vi "Actor Core.vi"(8 "error in":errorcluster, 11 "Guest Manager UI in":refnum<class "Guest Manager UI.lvclass">) -> (0 "error out":errorcluster, 3 "Actor out":refnum<class "Actor.lvclass">)   [LabVIEW 2023, in "Guest Manager UI.lvlib" / "Guest Manager UI.lvclass"]
doc: "(<B>Filename</B>: Actor Framework.lvlib:Actor.lvclass:Actor Core.vi)\n\nReceives messages to the actor, reacts to them, and initiates any error handling that may shut the actor down.\n\nDescendant classes may override this VI to append parallel tasks for the actor to complete while it handles messages. Overrides use the Call Parent Class Method node."
uses:
  Guest Manager UI.lvclass
  C:/Users/bhaghyaraj/Trainings/NI Actor Framework/SDLC/UI Base/UI Base/UI Base.lvclass
  C:/Program Files/National Instruments/LabVIEW 2023/vi.lib/ActorFramework/Actor/Actor.lvclass
  <vilib>/ActorFramework/Actor/Actor.lvclass
  Guest Manager UI.lvclass/Guest Manager UI.ctl
  <vilib>/ActorFramework/Actor/Actor.lvclass/Actor.ctl
  <vilib>/ActorFramework/Message Enqueuer/Message Enqueuer.lvclass/Message Enqueuer.ctl
  Guest Manager UI Messages/Check Guest History Msg/Check Guest History Msg.lvclass/Check Guest History Msg.ctl
  Guest Manager UI Messages/Fetch Rooms List and Size Limits Msg/Fetch Rooms List and Size Limits Msg.lvclass/Fetch Rooms List and Size Limits Msg.ctl
  Guest Manager UI Messages/Fetch Room Details Msg/Fetch Room Details Msg.lvclass/Fetch Room Details Msg.ctl
  <vilib>/ActorFramework/Message Enqueuer/Enqueue.vi
  <vilib>/ActorFramework/Message Enqueuer/Init from Existing Queue.vi
  <vilib>/ActorFramework/Stop Msg/Stop Msg.lvclass
  C:/Program Files/National Instruments/LabVIEW 2023/vi.lib/ActorFramework/Message/Message.lvclass
  Guest Manager UI Messages/Check Guest History Msg/Check Guest History Msg.lvclass
  Guest Manager UI Messages/Fetch Rooms List and Size Limits Msg/Fetch Rooms List and Size Limits Msg.lvclass
  Guest Manager UI Messages/Request Check-In Msg/Request Check-In Msg.lvclass
  Guest Manager UI Messages/Fetch Room Details Msg/Fetch Room Details Msg.lvclass
  Guest Manager UI Messages/Request Check-Out Msg/Request Check-Out Msg.lvclass
  Guest Manager UI Messages/Fetch Room Sizes Msg/Fetch Room Sizes Msg.lvclass
  <vilib>/ActorFramework/Message Priority Queue/Priority Enqueue.vi
  <vilib>/ActorFramework/Message Enqueuer/Message Enqueuer.lvclass
  UI Base/UI Base/UI Base.lvclass
  Utilities/Utilities.lvlib
panel:
  in  "Operation":enum32{"Check-In", "Check-Out"}(tab)
  in  "Children":u32=1 min=1
  in  "Primary Guest Name In":string caption="Primary Guest Name"
  in  "Guest Contact Number In":string caption="Guest Contact Number"
  in  "Room Size":u16(ring) items=["Suite (Non-AC)"]
  in  "Room Number In":u16(ring) caption="Room Number" items=["305"]
  in  "Adults":u32=1 min=1
  in  "Check-In":bool
  in  "Check-Out":bool
  out "Bill Summary":string
  out "Guest Contact Number Out":string caption="Guest Contact Number"
  out "Primary Guest Name Out":string caption="Primary Guest Name"
  out "Room Number Out":string caption="Room Number"
  # "Guest Check-In"
  # "Guest Check-Out"
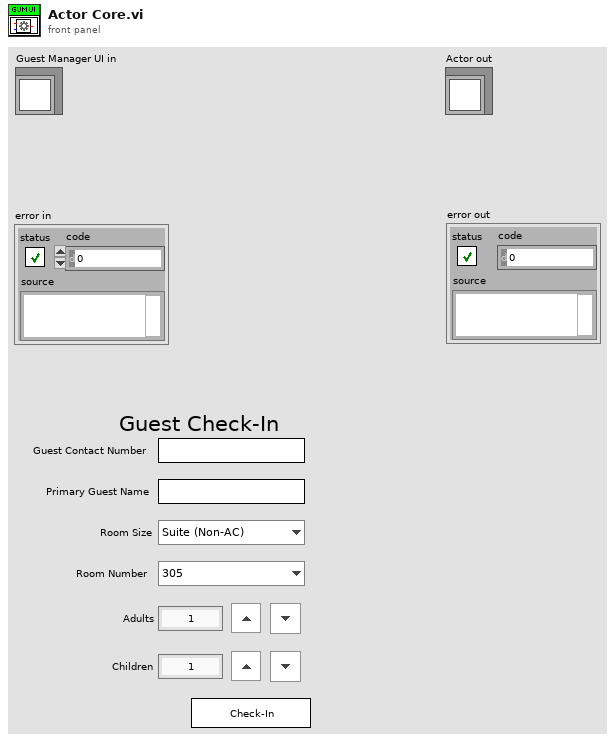
[diagram p1: front panel]
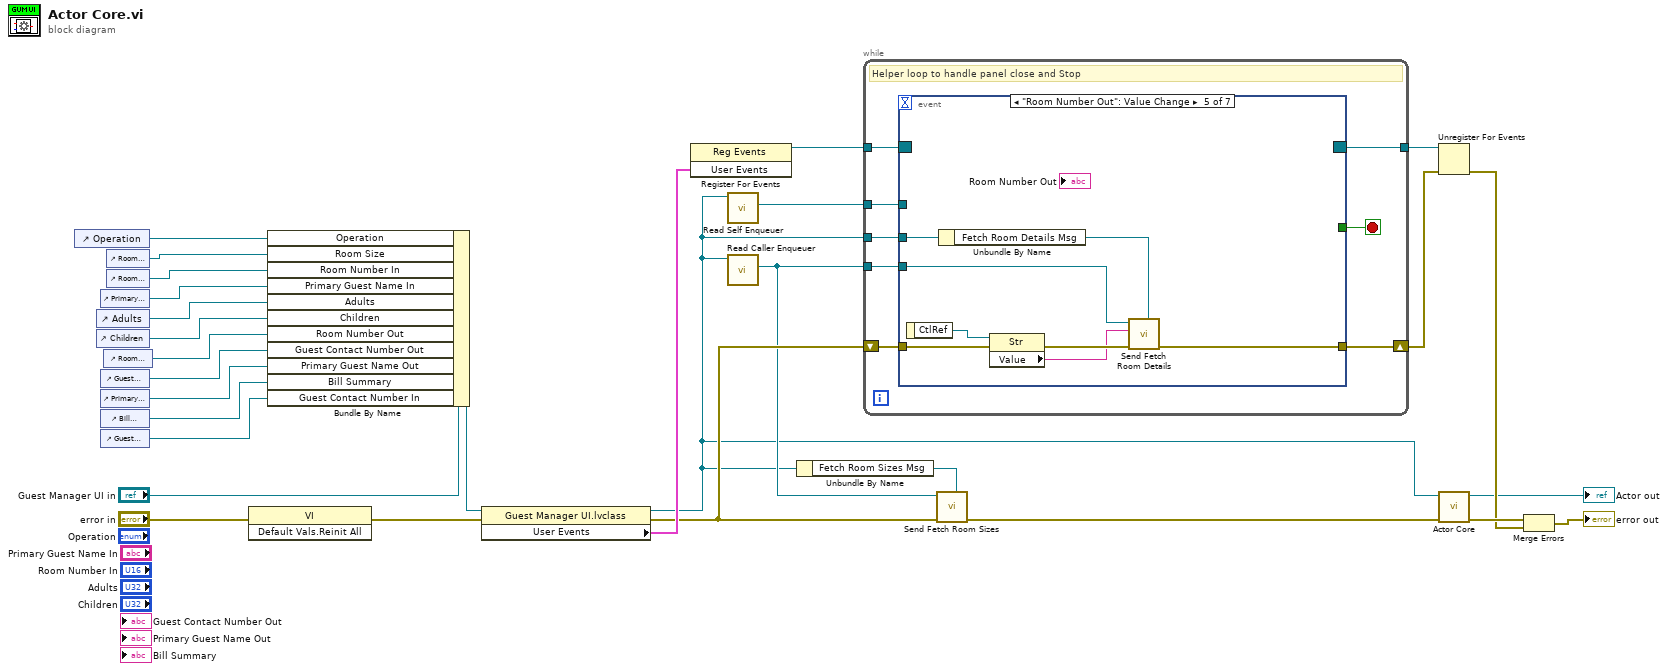
[diagram p0: block diagram]
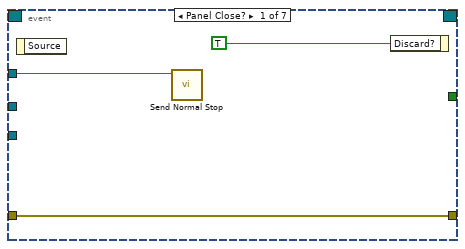
[diagram p2: hidden frame]
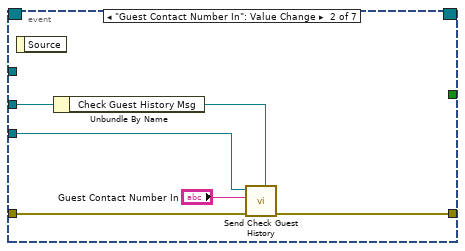
[diagram p3: hidden frame]
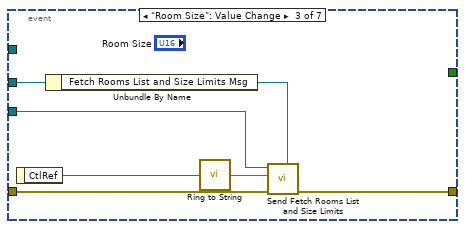
[diagram p4: hidden frame]
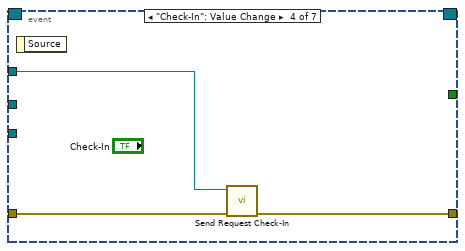
[diagram p5: hidden frame]
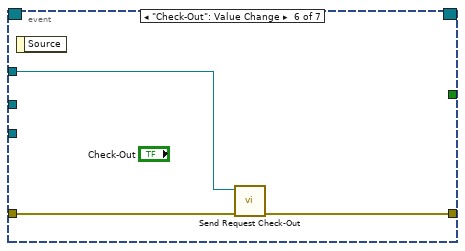
[diagram p6: hidden frame]
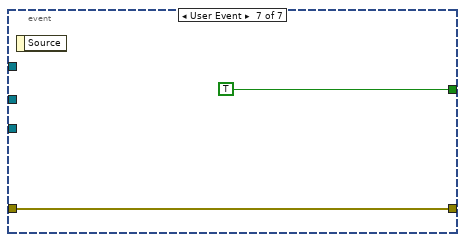
[diagram p7: hidden frame]
diagram:
  n1 = control-ref of="Operation"() -> (w17:refnum<vi>)
  n2 = control-ref of="Adults"() -> (w13:refnum<vi>)
  n3 = control-ref of="Children"() -> (w3:refnum<vi>)
  n4 = control-ref of="Primary Guest Name In"() -> (w14:refnum<vi>)
  n5 = control-ref of="Guest Contact Number Out"() -> (w11:refnum<vi>)
  n6 = control-ref of="Primary Guest Name Out"() -> (w10:refnum<vi>)
  n7 = control-ref of="Bill Summary"() -> (w9:refnum<vi>)
  n8 = control-ref of="Guest Contact Number In"() -> (w2:refnum<vi>)
  n9 = control-ref of="Room Number Out"() -> (w12:refnum<vi>)
  n10 = control-ref of="Room Size"() -> (w16:refnum<vi>)
  n11 = control-ref of="Room Number In"() -> (w15:refnum<vi>)
  n12 = invoke class="VI" method="Default Vals.Reinit All"(error in="error in") -> (error out=w1:errorcluster)  [unwired: 2 in, 2 out]
  n13 = Bundle By Name(cluster="Guest Manager UI in", "Operation"=w17, "Room Size"=w16, "Room Number In"=w15, "Primary Guest Name In"=w14, "Adults"=w13, "Children"=w3, "Room Number Out"=w12, "Guest Contact Number Out"=w11, "Primary Guest Name Out"=w10, "Bill Summary"=w9, "Guest Contact Number In"=w2) -> (w18:refnum<class "Guest Manager UI.lvclass">)
  n14 = property class="Guest Manager UI.lvclass"(reference=w18, error in=w1) -> (reference out=w5:refnum<class "Guest Manager UI.lvclass">, error out=w8:errorcluster, "User Events"=w25:cluster{"Stop":refnum<user-event>})
  n15 = register-events(w25) -> (reference out=w27:refnum<event-registration>)  [unwired: 2 in, 1 out]
  n16 = call <vilib>:"Read Self Enqueuer.vi"("Actor"=w5) -> ("Self Enqueuer"=w26:refnum<class "Message Enqueuer.lvclass">)  [unwired: 10 in]
  n17 = call <vilib>:"Read Caller Enqueuer.vi"("Actor"=w5) -> ("Caller Enqueuer"=w6:refnum<class "Message Enqueuer.lvclass">)  [unwired: 10 in]
  n18 = Unbundle By Name(w5) -> ("Fetch Room Sizes Msg"=w4:refnum<class "Fetch Room Sizes Msg.lvclass">)
  n19 = while {
    tunnel: w26 -> [w37]
    tunnel: w27 -> [w36]
    tunnel: [w34] -> w28
    tunnel: w6 -> [w33]
    tunnel: w5 -> [w32]
    shift-right: [w30] -> w23
    shift-left: w8 -> [w31]
    stop <- w35 stop-if-true
    # "Helper loop to handle panel close and Stop"
    n20 = event shown="[4] \"Room Number Out\": Value Change" {
      selector: w36 -> [_ _ _ _ _ _ _]
      dyn-events: [_ _ _ _ _ _ _] -> w34
      timeout: _ -> [_ _ _ _ _ _ _]
      tunnel: w37 -> [w39 _ _ w54 _ w65 _]
      tunnel: [_ _ _ _ _ _ TRUE] -> w35
      tunnel: w33 -> [_ w44 w51 _ w60 _ _]
      tunnel: w32 -> [_ w42 w50 _ w62 _ _]
      tunnel: w31 -> [w38 w46 w53 w56 w64 w67 w68]
      tunnel: [w38 w45 w52 w55 w63 w66 w68] -> w30
      event Panel Close? {
        n21 = event-data() -> ()  [unwired: 1 in, 1 out]
        n22 = call <vilib>:"Send Normal Stop.vi"("Message Enqueuer"=w39) -> ()  [unwired: 10 in, 1 out]
        n23 = event-data("Discard?"=TRUE) -> ()  [unwired: 1 in, 1 out]
      }
      event "Guest Contact Number In": Value Change {
        n24 = event-data() -> ()  [unwired: 1 in, 1 out]
        n25 = Unbundle By Name(w42) -> ("Check Guest History Msg"=w41:refnum<class "Check Guest History Msg.lvclass">)
        n26 = call "Send Check Guest History.vi"("Message Type"=w41, "error in (no error)"=w46, "Guest Contact Number In"="Guest Contact Number In", "Message Enqueuer"=w44) -> ("error out"=w45:errorcluster)  [unwired: 6 in, 1 out]
      }
      event "Room Size": Value Change {
        n27 = event-data() -> ("CtlRef"=w48:refnum<vi>)  [unwired: 1 in]
        n28 = Unbundle By Name(w50) -> ("Fetch Rooms List and Size Limits Msg"=w49:refnum<class "Fetch Rooms List and Size Limits Msg.lvclass">)
        n29 = call "Ring to String.vi"("Ring Ctrl Ref"=w48) -> ("Output String"=w47:string)
        n30 = call "Send Fetch Rooms List and Size Limits.vi"("Message Type"=w49, "error in (no error)"=w53, "Room Size"=w47, "Message Enqueuer"=w51) -> ("error out"=w52:errorcluster)  [unwired: 6 in, 1 out]
      }
      event "Check-In": Value Change {
        n31 = event-data() -> ()  [unwired: 1 in, 1 out]
        n32 = call "Send Request Check-In.vi"("error in (no error)"=w56, "Message Enqueuer"=w54) -> ("error out"=w55:errorcluster)  [unwired: 8 in, 1 out]
      }
      event "Room Number Out": Value Change {
        n33 = event-data() -> ("CtlRef"=w58:refnum<vi>)  [unwired: 1 in]
        n34 = Unbundle By Name(w62) -> ("Fetch Room Details Msg"=w61:refnum<class "Fetch Room Details Msg.lvclass">)
        n35 = property class="Str"(reference=w58, error in=w64) -> (error out=w59:errorcluster, "Value"=w57:string)  [unwired: 1 out]
        n36 = call "Send Fetch Room Details.vi"("Message Type"=w61, "error in (no error)"=w59, "Room No"=w57, "Message Enqueuer"=w60) -> ("error out"=w63:errorcluster)  [unwired: 6 in, 1 out]
      }
      event "Check-Out": Value Change {
        n37 = event-data() -> ()  [unwired: 1 in, 1 out]
        n38 = call "Send Request Check-Out.vi"("error in (no error)"=w67, "Message Enqueuer"=w65) -> ("error out"=w66:errorcluster)  [unwired: 8 in, 1 out]
      }
      event User Event {
        n39 = event-data() -> ()  [unwired: 1 in, 1 out]
      }
    }
  }
  n40 = call "Send Fetch Room Sizes.vi"("Message Type"=w4, "error in (no error)"=w8, "Message Enqueuer"=w6) -> ("error out"=w7:errorcluster)  [unwired: 7 in, 1 out]
  n41 = Unregister For Events(event registration refnum=w28, error in=w23) -> (error out=w24:errorcluster)
  n42 = call-parent "Actor Core.vi"("error in"=w7, "Actor in"=w5) -> ("error out"=w29:errorcluster, "Actor out"=→"Actor out":refnum<class "Actor.lvclass">)  [unwired: 8 in]
  n43 = Merge Errors(w29, w24) -> (→"error out":errorcluster)
